vi "ProdaNG.Configurator.Glb.Write.vi"(7 "DB":T1, 8 "error in (no error)":errorcluster) -> (0 "error out":errorcluster)   [LabVIEW 2016]
uses:
  ProdaNG.Configurator.DB.ctl
  Tools/Tma.lib/nlconfig.llb/fp2ini mode.ctl
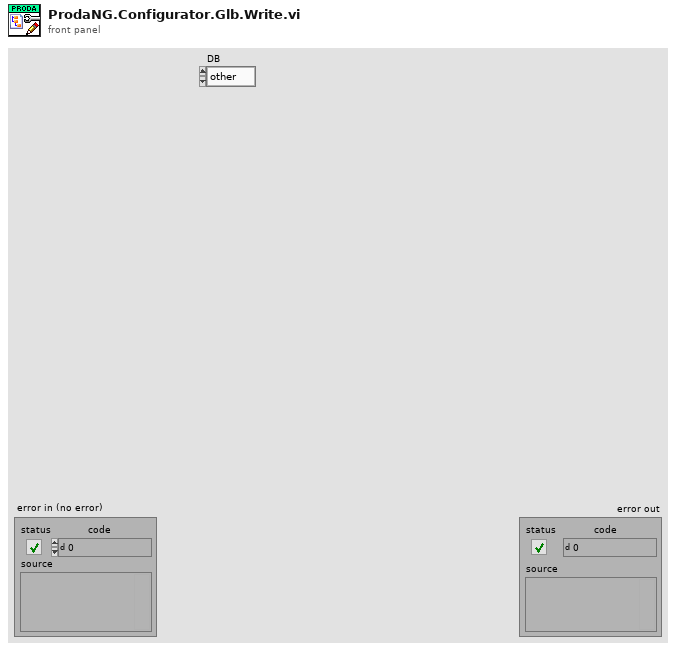
[diagram p1: front panel]
types:
  T1 = typedef "ProdaNG.Configurator.DB.ctl" = enum16{"other", "WPL", "WPK"}
  T2 = typedef "fp2ini mode.ctl" = enum16{"Read Controls", "Write Controls", "Write Indicators", "Read Indicators", "Write all", "Read all"}
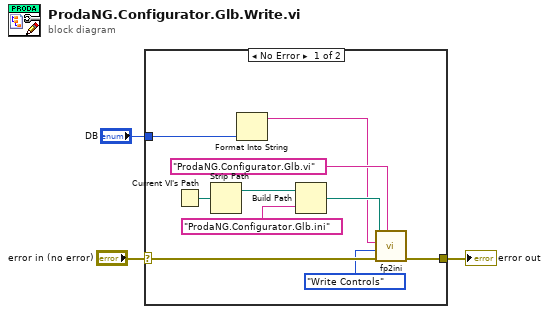
[diagram p0: block diagram]
diagram:
  n1 = case shown="No Error" "error in (no error)" {
    selector: "error in (no error)" -> [w8 w14]
    tunnel: [w5 w14] -> w2
    tunnel: "DB" -> [w7 _]
    frame No Error {
      n2 = Current VI's Path() -> (path=w13:path)
      n3 = Strip Path(path=w13) -> (stripped path=w12:path)  [unwired: 1 out]
      n4 = Format Into String(w7) -> (resulting string=w6:string)  [unwired: 3 in, 1 out]
      n5 = Build Path(base path=w12, name or relative path="ProdaNG.Configurator.Glb.ini") -> (appended path=w9:path)
      n6 = call "fp2ini.vi"("vi-name (caller if empty)"="ProdaNG.Configurator.Glb.vi" ("name or relative path"), "error in"=w8, "mode"=fp2ini_mode."Write Controls", "section"=w6, "ini-file path"=w9) -> ("error out"=w5:errorcluster)  [unwired: 6 in]
    }
    frame Error {
    }
  }
  "error out" <- w2
